vi "frame-input-engine.vi"(8 "error in (no error)":errorcluster, 9 "CAN Cluster":refnum<k21>=":memory:", 10 "Select Interface":refnum<k21>="CAN2", 11 "frameQ":refnum<queue>) -> ()   [LabVIEW 2015]
doc: "This example demonstrates frame streaming input using an NI-XNET Frame Input session. \n\nThis example can run against any output example, assuming you have a properly terminated CAN cable connected to two CAN ports.\n\nIf you have no database aliases on your system, the example automatically loads the nixnet_example database."
uses:
  <vilib>/ErrorRing/Error Ring.xnode
  <vilib>/Utility/error.llb/Error Cluster From Error Code.vi
  <vilib>/xnet/xnet.llb/XNET Read (Frame CAN).vi
  <vilib>/xnet/xnet.llb/XNET Create Session (Frame Input Stream).vi
  <vilib>/xnet/xnet.llb/XNET Frame Type CAN.ctl
  <vilib>/xnet/xnet.llb/XNET Frame CAN.ctl
panel:
  out "error out":errorcluster
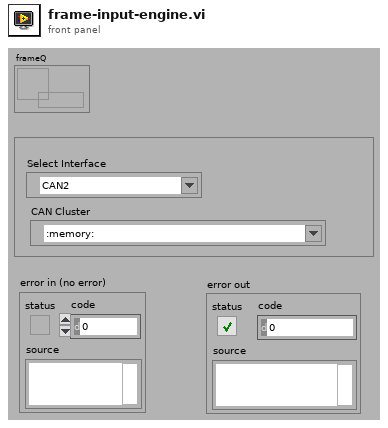
[diagram p1: front panel]
types:
  T1 = typedef "CAN_FRAME.ctl" = cluster{"timestamp":timestamp, "payload":u8[], "identifier":u32, "type":T2, "extended?":bool, "echo?":bool, "payload.len":u8}
  T2 = typedef "XNET Frame Type CAN.ctl" = u8
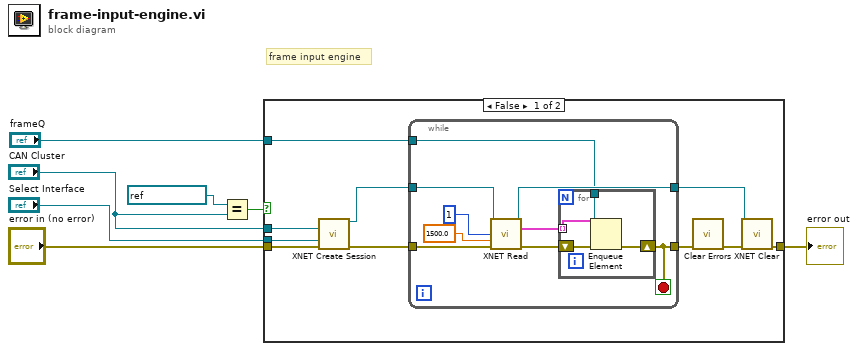
[diagram p0: block diagram]
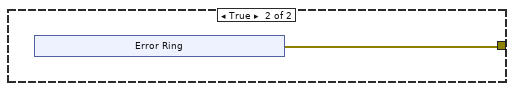
[diagram p2: hidden frame]
diagram:
  # "frame input engine"
  n1 = Equal?(x=refnum<k21> ":memory:" ("CAN Cluster"), y="CAN Cluster") -> (x = y?=w2:bool)
  n2 = case shown="False" w2 {
    tunnel: "Select Interface" -> [w17 _]
    tunnel: "CAN Cluster" -> [w16 _]
    tunnel: "error in (no error)" -> [w15 _]
    tunnel: [w13 w31] -> w3
    tunnel: "frameQ" -> [w8 _]
    frame False {
      n3 = call-poly <vilib>:"XNET Create Session.vi"("cluster (:memory:)"=w16, "interface"=w17, "error in (no error)"=w15) -> ("session out"=w10:refnum<k21>, "error out"=w11:errorcluster)  [unwired: 11 out]
      n4 = while {
        tunnel: w10 -> [w26]
        tunnel: w11 -> [w25]
        tunnel: [w21] -> w14
        tunnel: [w20] -> w12
        tunnel: w8 -> [w18]
        stop <- w21 stop-if-true
        n5 = call-poly <vilib>:"XNET Read.vi"("session in"=w26, "number to read (-1)"=1, "timeout (0)"=1500.0, "error in (no error)"=w25) -> ("session out"=w20:refnum<k21>, "data"=w19:T1[], "error out"=w22:errorcluster)  [unwired: 9 out]
        n6 = for {
          shift-right: [w29] -> w21
          shift-left: w22 -> [w30]
          tunnel: w19 -> [w28] mode=indexing
          tunnel: w18 -> [w27]
          n7 = Enqueue Element(queue=w27, element=w28, error in (no error)=w30) -> (error out=w29:errorcluster)  [unwired: 1 in, 2 out]
        }
      }
      n8 = call <vilib>:"Clear Errors.vi"("error in (no error)"=w14) -> ("error out"=w9:errorcluster)  [unwired: 5 in, 1 out]
      n9 = call <vilib>:"XNET Clear.vi"("session in"=w12, "error in (no error)"=w9) -> ("error out"=w13:errorcluster)  [unwired: 13 in]
    }
    frame True {
      n10 = xnode "Error Ring"() -> ("error out"=w31:errorcluster)
    }
  }
  "error out" <- w3
